vi "Write GUI Events.vi"(8 "Error In":errorcluster, 10 "GUI Events":T1, 11 "BNT_SLTagMonitor in":refnum<class "BNT_SLTagMonitor.lvclass">) -> (0 "Error Out":errorcluster, 3 "BNT_SLTagMonitor out":refnum<class "BNT_SLTagMonitor.lvclass">)   [LabVIEW 2019, in "BNT_SLTagMonitor.lvlib" / "BNT_SLTagMonitor.lvclass"]
doc: "Write GUI event references to attribute."
uses:
  BNT_SLTagMonitor.lvclass
  CSPP_Core/Messages/CSPP_PVUpdate Msg/CSPP_PVUpdate Msg.lvclass
  <vilib>/ActorFramework/Message Enqueuer/Message Enqueuer.lvclass
  <vilib>/Skyline/Tag/Wrapper/Wrapper_class/NI Skyline Tag.lvclass
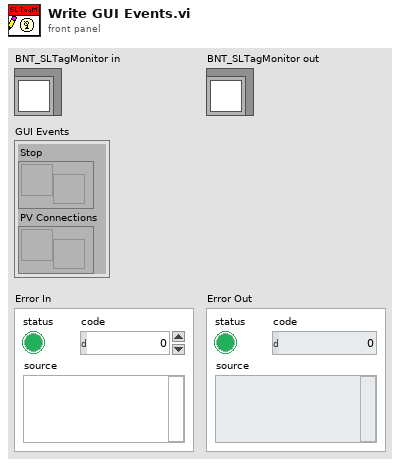
[diagram p1: front panel]
types:
  T1 = cluster{"Stop":refnum<user-event>, "PV Connections":refnum<user-event>}
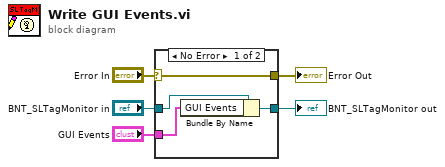
[diagram p0: block diagram]
diagram:
  n1 = case shown="No Error" "Error In" {
    selector: "Error In" -> [w9 w10]
    tunnel: [w9 w10] -> w1
    tunnel: [w7 w11] -> w4
    tunnel: "BNT_SLTagMonitor in" -> [w8 w11]
    tunnel: "GUI Events" -> [w6 _]
    frame No Error {
      n2 = Bundle By Name(cluster=w8, "GUI Events"=w6) -> (w7:refnum<class "BNT_SLTagMonitor.lvclass">)
    }
    frame Error {
    }
  }
  "BNT_SLTagMonitor out" <- w4
  "Error Out" <- w1
